vi "ReadManyChannels.vi"() -> ()   [LabVIEW 2021, in "XNET-CAN-Signal-Logger.lvlib"]
uses:
  <vilib>/xnet/xnet.llb/XNET Create Session (Signal Input Waveform).vi
  <vilib>/xnet/xnet.llb/XNET Read (Signal Waveform) .vi
  XNET-CAN-Signal-Logger.lvlib
  <resource>/objmgr/xnet.rc
panel:
  out "Queue Size":u32
  out "Num Signals":i32
  out "Av Samples/sec":dbl
  out "error out":errorcluster
  out "Samples Rd":i32
  in  "stop":bool
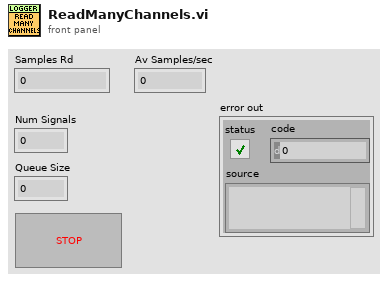
[diagram p1: front panel]
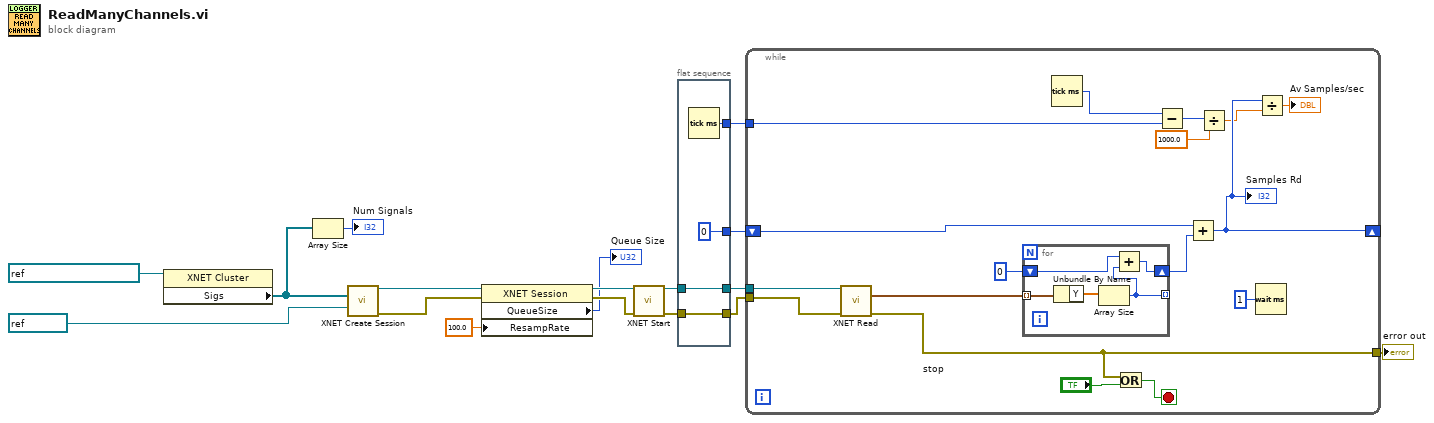
[diagram p0: block diagram]
diagram:
  n1 = property class="XNET Cluster"(reference=refnum<k21> "ManyXnetChannels" ("XNET Cluster")) -> ("Sigs"=w9:refnum<k21>[])  [unwired: 1 in, 2 out]
  n2 = Array Size(array=w9) -> (size(s)=→"Num Signals":i32)
  n3 = call-poly <vilib>:"XNET Create Session.vi"("signal list"=w9, "interface"=refnum<k21> "CAN1") -> ("session out"=w15:refnum<k21>, "error out"=w14:errorcluster)  [unwired: 12 in]
  n4 = property class="XNET Session"(reference=w15, error in=w14, "ResampRate"=100.0 ("Resample Rate")) -> (reference out=w7:refnum<k21>, error out=w6:errorcluster, "QueueSize"=→"Queue Size":u32)
  n5 = call <vilib>:"XNET Start.vi"("session in"=w7, "error in (no error)"=w6) -> ("session out"=w3:refnum<k21>, "error out"=w5:errorcluster)  [unwired: 12 in]
  n6 = flat-sequence {
    tunnel: [0 ("size(s)")] -> w12
    tunnel: [w20] -> w11
    tunnel: w5 -> [w19]
    tunnel: [w19] -> w4
    tunnel: w3 -> [w18]
    tunnel: [w18] -> w2
    frame #0 {
      n7 = Tick Count (ms)() -> (millisecond timer value=w20:u32)
    }
  }
  n8 = while {
    tunnel: w2 -> [w38]
    tunnel: w4 -> [w37]
    shift-right: [w24] -> _
    shift-left: w12 -> [w33]
    tunnel: w11 -> [w27]
    tunnel: [w29] -> w10
    stop <- w35 stop-if-true
    n9 = call-poly <vilib>:"XNET Read.vi"("session in"=w38, "error in (no error)"=w37) -> ("data"=w32:waveform(dbl)[], "error out"=w29:errorcluster)  [unwired: 11 in, 1 out]
    n10 = for {
      tunnel: w32 -> [w43] mode=indexing
      tunnel: [w41] -> _ mode=indexing
      shift-right: [w39] -> w30
      shift-left: 0 ("size(s)") -> [w40]
      n11 = Unbundle By Name(w43) -> ("Y"=w42:dbl[])
      n12 = Array Size(array=w42) -> (size(s)=w41:i32)
      n13 = Add(x=w40, y=w41) -> (x+y=w39:i32)
    }
    n14 = Tick Count (ms)() -> (millisecond timer value=w28:u32)
    n15 = Or(x=w29, y="stop") -> (x .or. y?=w35:bool)
    n16 = Subtract(x=w28, y=w27) -> (x-y=w26:u32)
    n17 = Add(x=w33, y=w30) -> (x+y=w24:i32)
    "Samples Rd" <- w24
    n18 = Divide(x=w26, y=1000.0) -> (x/y=w23:dbl)
    n19 = Wait (ms)(milliseconds to wait=u32 1) -> ()  [unwired: 1 out]
    n20 = Divide(x=w24, y=w23) -> (x/y=→"Av Samples/sec":dbl)
  }
  "error out" <- w10
